vi "Set Mode.vi"(8 "error in (no error)":errorcluster, 10 "New Mode":T1, 11 "Application in":refnum<class "Application.lvclass">) -> (0 "error out":errorcluster, 3 "Application out":refnum<class "Application.lvclass">)   [LabVIEW 2018, in "Application.lvlib" / "Application.lvclass"]
uses:
  Application.lvclass
  Mode.ctl
  Application.lvclass/Application.ctl
  User Interface/Main Window Messages/Application Mode Change Msg/Application Mode Change Msg.lvclass/Application Mode Change Msg.ctl
  <vilib>/ActorFramework/Message Enqueuer/Message Enqueuer.lvclass/Message Enqueuer.ctl
  <vilib>/ActorFramework/Message Enqueuer/Enqueue.vi
  User Interface/Main Window Messages/Application Mode Change Msg/Application Mode Change Msg.lvclass
  C:/Program Files/National Instruments/LabVIEW 2018/vi.lib/ActorFramework/Message/Message.lvclass
  <vilib>/ActorFramework/Message Priority Queue/Priority Enqueue.vi
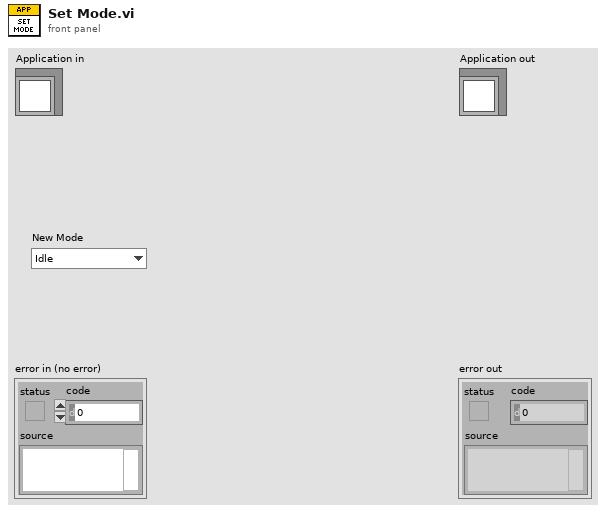
[diagram p1: front panel]
types:
  T1 = typedef "Mode.ctl" = enum16{"Idle", "Cancel", "Live", "Stream", "Autofocus", "Z-Stack"}
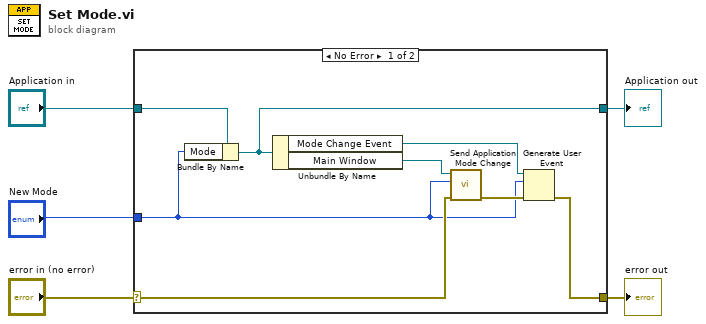
[diagram p0: block diagram]
diagram:
  n1 = case shown="No Error" "error in (no error)" {
    selector: "error in (no error)" -> [w10 w15]
    tunnel: [w8 w15] -> w4
    tunnel: [w12 w14] -> w2
    tunnel: "Application in" -> [w13 w14]
    tunnel: "New Mode" -> [w6 _]
    frame No Error {
      n2 = Bundle By Name(cluster=w13, "Mode"=w6) -> (w12:refnum<class "Application.lvclass">)
      n3 = Unbundle By Name(w12) -> ("Mode Change Event"=w7:refnum<user-event>, "Main Window"=w11:refnum<class "Message Enqueuer.lvclass">)
      n4 = call "Send Application Mode Change.vi"("error in (no error)"=w10, "Mode"=w6, "Message Enqueuer"=w11) -> ("error out"=w9:errorcluster)  [unwired: 7 in, 1 out]
      n5 = Generate User Event(user event=w7, event data cluster=w6, error in=w9) -> (error out=w8:errorcluster)  [unwired: 1 in, 1 out]
    }
    frame Error {
    }
  }
  "error out" <- w4
  "Application out" <- w2
